vi "ANN.vi"(0 "Input":dbl[](array[numeric])=[2.0, 4.0, -2.0], 1 "Iterations":i32(slide)=1 scale=0.0..500.0, 3 "Beta":dbl(slide)=1.0 scale=0.0..4.0, 5 "Target Output":dbl[](array[numeric])=[1.0, 1.0, 0.0, 1.0], 7 "Weight_2":dbl[][](array[numeric])=[[0.8370162109753583, -0.4589512757043748, -0.9209152655432105, 0.22980134575141165], [-0.3076334000925458, 0.3779075166237016, -0.7121350594088285, 0.5657425254894664], [-0.37857381518782107, 0.4595383310211245, -0.4040891935767137, 0.8618781458120324], [0.1, 0.1, 0.1, 0.1]], 9 "Weight_1":dbl[][](array[numeric])=[[0.22641122957224669, 0.9000532537551416, -0.6893260062220201, -0.891456684225945], [0.76528437998916, 0.16167194121278605, 0.6328018015855013, 0.9526181449019115], [0.20556072382043, -0.2917865013532386, 0.08921931448581022, -0.29348885779366407], [0.2189626962972664, -0.5938027052670742, -0.7920590296764609, -0.5253766022852844]], 11 "Back Propagation":bool, 12 "Learning Rate":dbl(slide)=0.49999999999999994 scale=0.0..1.0) -> (4 "output":dbl[](array[slide]) scale=0.0..1.0, 10 "Weight_2_out":dbl[][](array[numeric]), 14 "Weight_1_out":dbl[][](array[numeric]), 15 "Error":dbl(graph))   [LabVIEW 2009]
uses:
  <vilib>/Analysis/_algsub.llb/Real Vector Norm.vi
  <vilib>/Analysis/NI_AALPro.lvlib
panel:
  out "End layer weight":dbl[][](array[numeric])
  out "First layer weight":dbl[][](array[numeric])
  # "bias node = -1 is automatically incorporated. Don't forget to include the weights for it (dimensions should agree accordingly)"
  # "must include bias node for the input for each node for the weights"
  # "input"
  # "input"
  # "output"
  # "output"
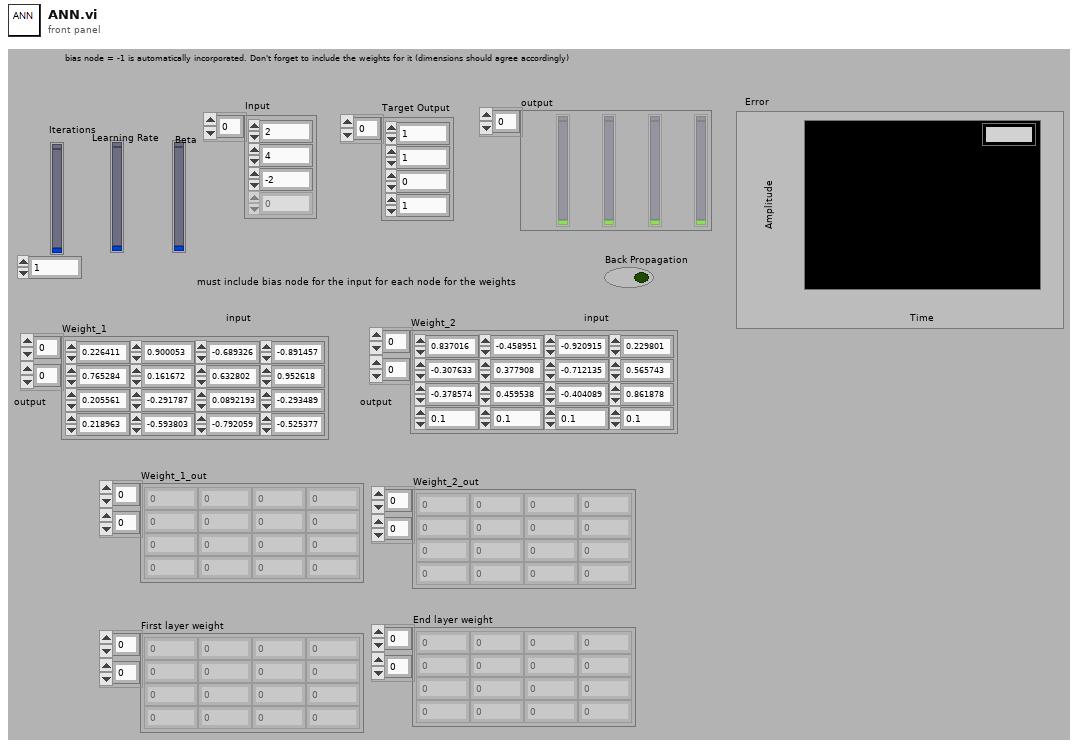
[diagram p1: front panel]
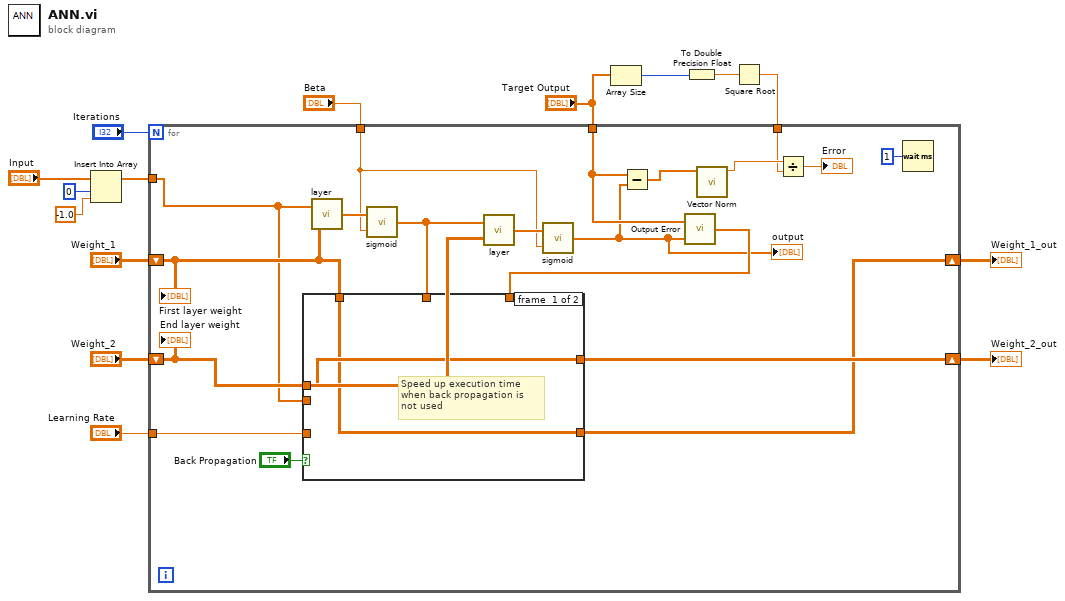
[diagram p0: block diagram]
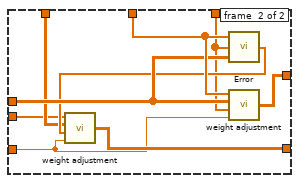
[diagram p2: hidden frame]
diagram:
  n1 = Insert Into Array(array="Input", index=0, new element=-1.0 ("new element/subarray")) -> (w9:dbl[])
  n2 = Array Size(array="Target Output") -> (size(s)=w2:i32)
  n3 = To Double Precision Float(number=w2) -> (double precision float=w1:dbl)
  n4 = Square Root(x=w1) -> (sqrt(x)=w3:dbl)
  n5 = for {
    N: "Iterations" -> [_]
    tunnel: w9 -> [w24]
    shift-right: [w30] -> w13
    shift-left: "Weight_2" -> [w31]
    shift-right: [w28] -> w14
    shift-left: "Weight_1" -> [w29]
    tunnel: "Learning Rate" -> [w26]
    tunnel: "Target Output" -> [w22]
    tunnel: "Beta" -> [w21]
    tunnel: w3 -> [w19]
    n6 = call "layer.vi"("weight"=w29, "Input"=w24) -> ("Output"=w34:dbl[])
    n7 = call "sigmoid.vi"("Beta"=w21, "input"=w34) -> ("output"=w32:dbl[])
    n8 = call "layer.vi"("weight"=w31, "Input"=w32) -> ("Output"=w33:dbl[])
    n9 = call "sigmoid.vi"("Beta"=w21, "input"=w33) -> ("output"=w17:dbl[])
    "output" <- w17
    n10 = Subtract(x=w22, y=w17) -> (x-y=w23:dbl[])
    n11 = call "Output Error.vi"("Output"=w17, "Target Output"=w22) -> ("End Error"=w25:dbl[])
    n12 = case shown="True" "Back Propagation" {
      tunnel: w32 -> [_ w45]
      tunnel: w31 -> [w36 w44]
      tunnel: [w36 w43] -> w30
      tunnel: w29 -> [w35 w41]
      tunnel: [w35 w40] -> w28
      tunnel: w26 -> [_ w39]
      tunnel: w25 -> [_ w38]
      tunnel: w24 -> [_ w37]
      frame #0 {
        # "Speed up execution time when back propagation is not used"
      }
      frame #1 {
        n13 = call "Error.vi"("Weight"=w44, "Forward Error"=w38, "Output"=w45) -> ("Out Error"=w42:dbl[])
        n14 = call "weight adjustment.vi"("Learning Rate"=w39, "Error"=w42, "Weight"=w41, "Input"=w37) -> ("Weight out"=w40:dbl[][])
        n15 = call "weight adjustment.vi"("Learning Rate"=w39, "Error"=w38, "Weight"=w44, "Input"=w45) -> ("Weight out"=w43:dbl[][])
      }
    }
    n16 = call-poly <vilib>:"Vector Norm.vi"("Input Vector"=w23) -> ("norm"=w20:dbl)  [unwired: 9 in, 1 out]
    n17 = Divide(x=w20, y=w19) -> (x/y=→"Error":dbl)
    n18 = Wait (ms)(milliseconds to wait=u32 1) -> ()  [unwired: 1 out]
    "First layer weight" <- w29
    "End layer weight" <- w31
  }
  "Weight_1_out" <- w14
  "Weight_2_out" <- w13
